vi "niDTS WLAN INSTR TX Close.vi"(8 "error in (no error)":errorcluster, 11 "niDTS WLAN INSTR TX in":refnum<class "niDTS WLAN INSTR TX.lvclass">) -> (0 "error out":errorcluster)   [LabVIEW 2015, in "niDTS WLAN.lvlib" / "niDTS WLAN INSTR TX.lvclass"]
uses:
  niDTS WLAN INSTR TX.lvclass
  niDTS WLAN INSTR TX.lvclass/niDTS WLAN INSTR TX.ctl
  RiviInstDriver/InstDriver/Objects/InstDriver.lvclass
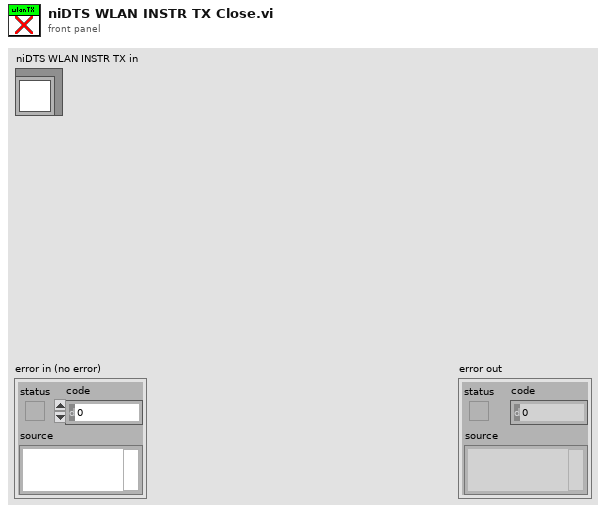
[diagram p1: front panel]
types:
  T1 = typedef "niRfsaWlan.lvclass/niRfsaWlan INC Handle.ctl" = refnum<data-value>
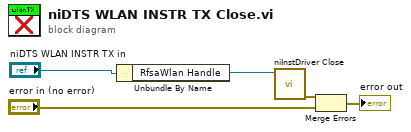
[diagram p0: block diagram]
diagram:
  n1 = Unbundle By Name("niDTS WLAN INSTR TX in") -> ("RfsaWlan Handle"=w3:T1)
  n2 = call "niInstDriver Close.vi"("InstDriver Handle in"=w3) -> ("error out"=w2:errorcluster)  [unwired: 14 in]
  n3 = Merge Errors(w2, "error in (no error)") -> (→"error out":errorcluster)
